vi "Dialog_LogMeas (SubVI).vi"() -> ()   [LabVIEW 2017]
uses:
  <vilib>/Utility/miscctls.llb/LVRowAndColumnTypeDef.ctl
  Global_SNK3_HF.vi
panel:
  in  "ToExcelTableMeas":bool
  in  "ClearTableMeas":bool
  in  "AddToTable":bool
  out "TableMeas":string[][](table)
  in  "Enum":enum16{"ПЭП 1...8", "ПЭП 9...16"}(ring) caption="Запись в таблицу"
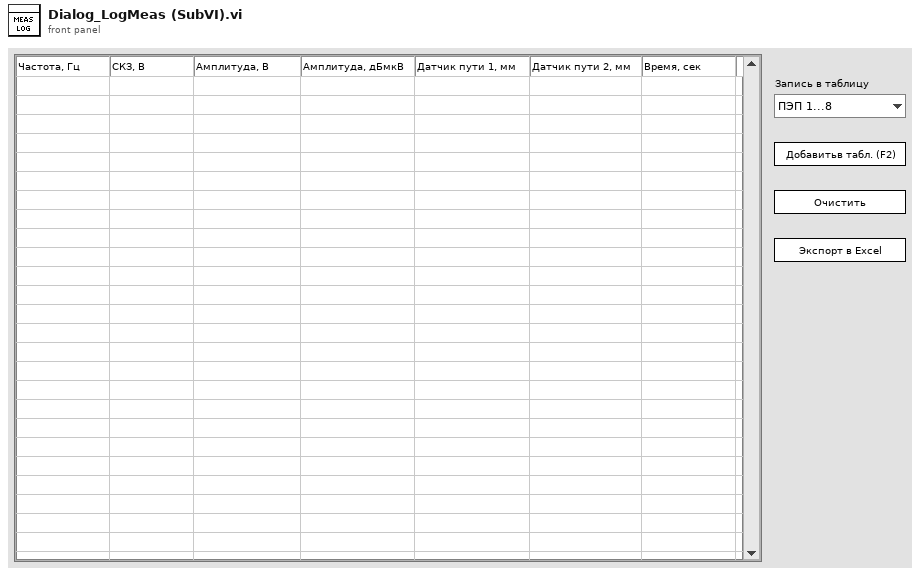
[diagram p1: front panel]
types:
  T1 = typedef "LVRowAndColumnTypeDef.ctl" = cluster{"Row":i32, "Column":i32}
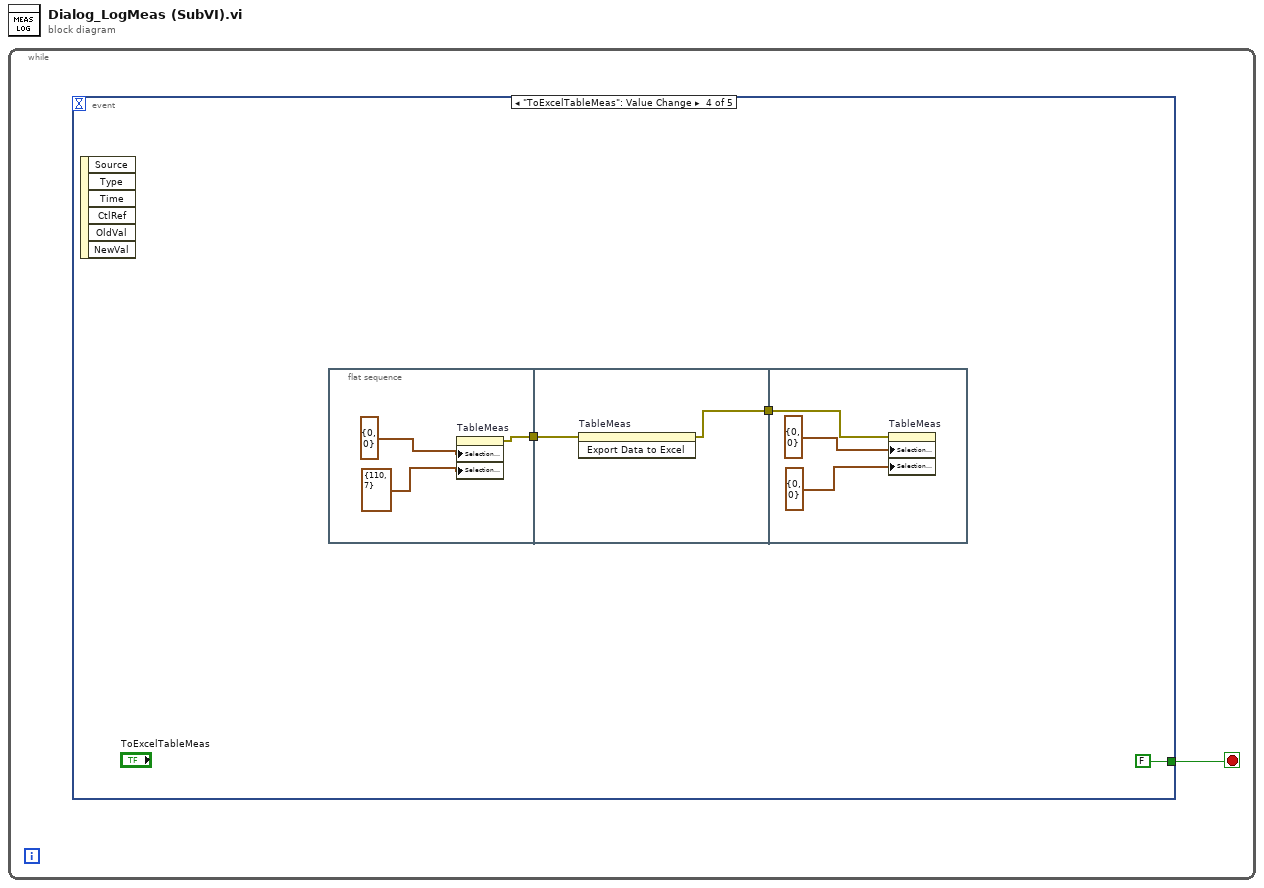
[diagram p0: block diagram]
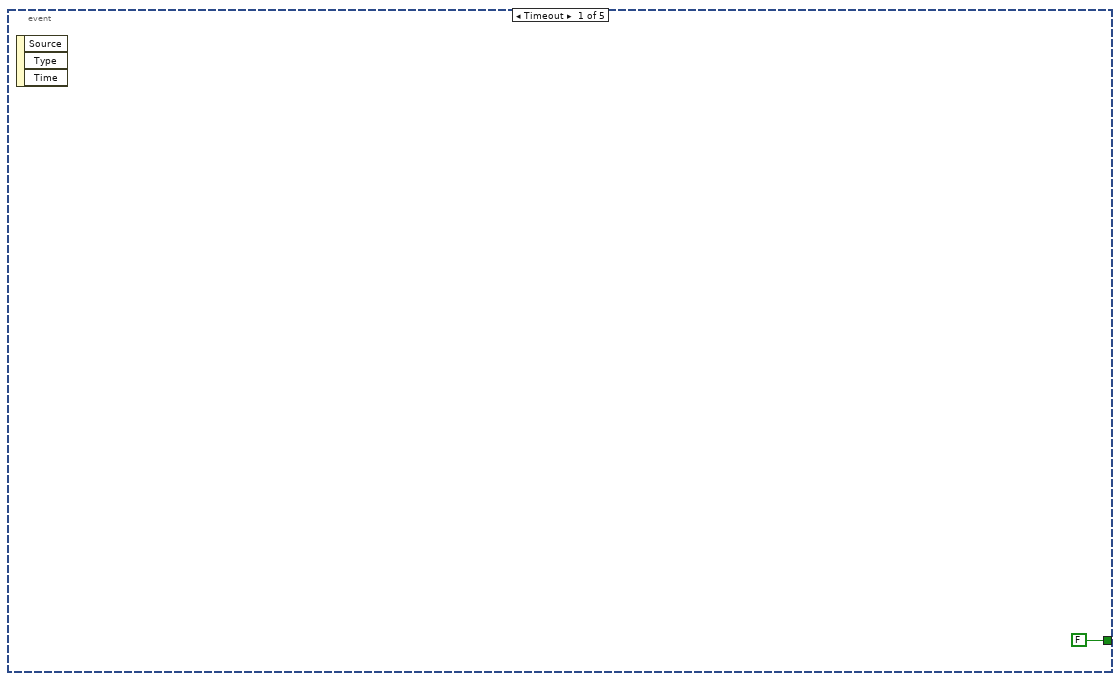
[diagram p2: hidden frame]
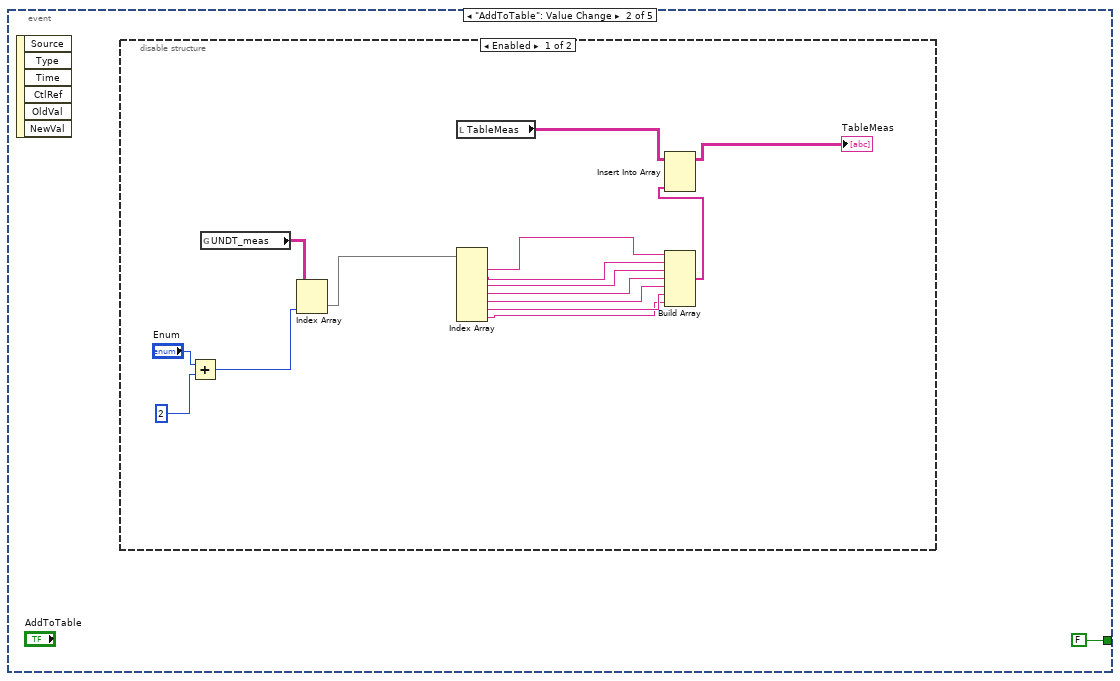
[diagram p3: hidden frame]
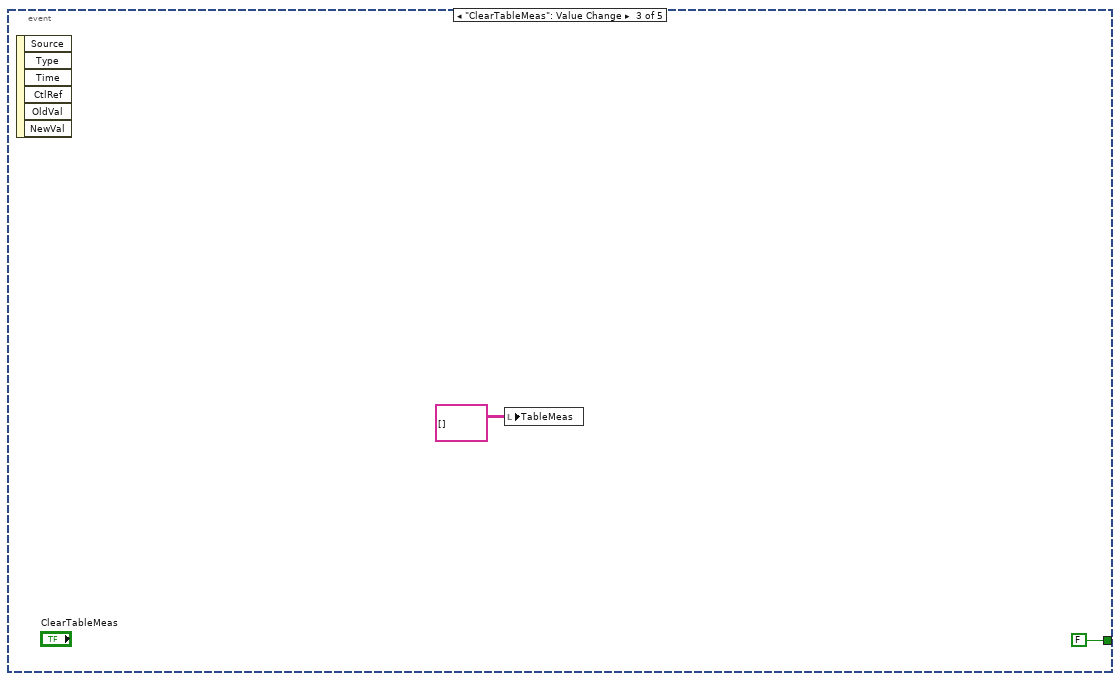
[diagram p5: hidden frame]
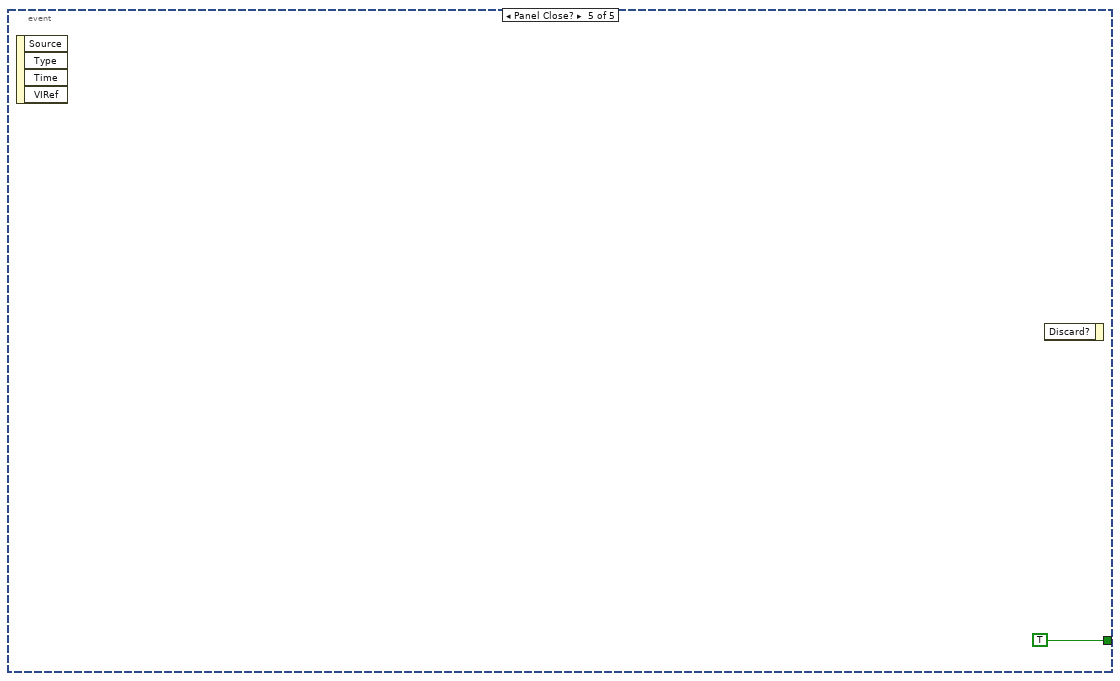
[diagram p6: hidden frame]
diagram:
  n1 = while {
    stop <- w1 stop-if-true
    n2 = event shown="[3] \"ToExcelTableMeas\": Value Change" {
      selector: _ -> [_ _ _ _ _]
      dyn-events: _ -> [_ _ _ _ _]
      timeout: _ -> [_ _ _ _ _]
      tunnel: [FALSE FALSE FALSE FALSE TRUE] -> w1
      event Timeout {
        n3 = event-data() -> ()  [unwired: 1 in, 3 out]
      }
      event "AddToTable": Value Change {
        n4 = event-data() -> ()  [unwired: 1 in, 6 out]
        n5 = disable-structure shown="Enabled" {
          frame Enabled {
            n6 = Add(x="Enum", y=2) -> (x+y=w12:i32)
            n7 = global read "Global_SNK3_HF.vi" "UNDT_meas"() -> (w15:string[][])
            n8 = Index Array(array=w15, index (col)=w12) -> (element=w11:string[])  [unwired: 1 in]
            n9 = local read "TableMeas"() -> (w18:string[][])
            n10 = Index Array(array=w11) -> (element #1=w10:string, element #2=w9:string, element #3=w8:string, element #4=w7:string, element #5=w6:string, element #6=w5:string, element #7=w4:string)  [unwired: 7 in]
            n11 = Build Array(w10, w9, w8, w7, w6, w5, w4) -> (w16:string[])
            n12 = Insert Into Array(array=w18, new element=w16) -> (→"TableMeas":string[][])  [unwired: 2 in]
          }
          frame Disabled {
          }
        }
      }
      event "ClearTableMeas": Value Change {
        n13 = event-data() -> ()  [unwired: 1 in, 6 out]
        n14 = local write "TableMeas"(string[][] [] ("TableMeas")) -> ()
      }
      event "ToExcelTableMeas": Value Change {
        n15 = event-data() -> ()  [unwired: 1 in, 6 out]
        n16 = flat-sequence {
          tunnel: [w24] -> w22
          tunnel: w22 -> [w28]
          tunnel: [w27] -> w21
          tunnel: w21 -> [w31]
          frame #0 {
            n17 = property on="TableMeas" class="Tbl (strict)"("Selection Start"=T1 {"Row"=0, "Column"=0} ("Active Cell:Active Cell"), "Selection Size"=T1 {"Row"=110, "Column"=7}) -> (error out=w24:errorcluster)  [unwired: 2 in, 1 out]
          }
          frame #1 {
            n18 = invoke on="TableMeas" class="Tbl (strict)" method="Export Data to Excel"(error in=w28) -> (error out=w27:errorcluster)  [unwired: 2 in, 2 out]
          }
          frame #2 {
            n19 = property on="TableMeas" class="Tbl (strict)"(error in=w31, "Selection Start"=T1 {"Row"=0, "Column"=0} ("Active Cell:Active Cell"), "Selection Size"=T1 {"Row"=0, "Column"=0}) -> ()  [unwired: 1 in, 2 out]
          }
        }
      }
      event Panel Close? {
        n20 = event-data() -> ()  [unwired: 1 in, 4 out]
        n21 = event-data() -> ()  [unwired: 2 in, 1 out]
      }
    }
  }
